vi "init_calibration_arrays.vi"(9 "increment":dbl, 10 "start point":dbl, 11 "end point":dbl) -> (1 "number of points":dbl, 3 "initialized arrays":cluster{dbl[], dbl[]})   [LabVIEW 2015]
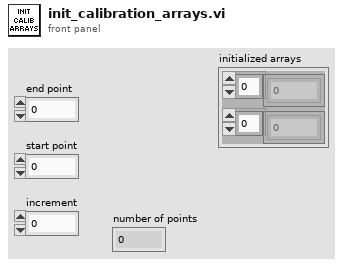
[diagram p1: front panel]
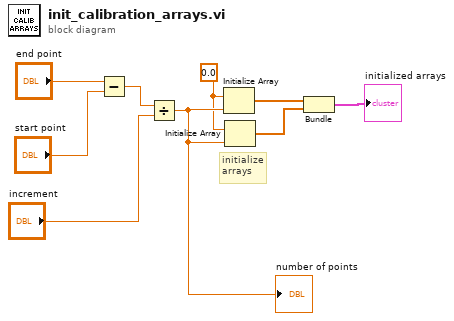
[diagram p0: block diagram]
diagram:
  w5 = 0.0 ("element")
  # "initialize\narrays"
  n1 = Subtract(x="end point", y="start point") -> (x-y=w4:dbl)
  n2 = Divide(x=w4, y="increment") -> (x/y=w8:dbl)
  "number of points" <- w8
  n3 = Initialize Array(w5, w8) -> (w3:dbl[])
  n4 = Initialize Array(w5, w8) -> (w2:dbl[])
  n5 = Bundle(w3, w2) -> (→"initialized arrays":cluster{dbl[], dbl[]})  [unwired: 1 in]
